vi "S4GUI.vi"() -> ()   [LabVIEW 2018] (continued)
        n3145 = call-dynamic "Read AcquisitionA.vi"("error in (no error)"=w7567, "S4ACS_GUI in"=w7556) -> ("error out"=w7581:errorcluster, "Acquisition.lvclass"=w7582:refnum<class "Acquisition.lvclass">)  [unwired: 7 in, 1 out]
        n3146 = call "Read AcquisitionB.vi"("error in (no error)"=w7567, "S4ACS_GUI in"=w7556) -> ("error out"=w7579:errorcluster, "Acquisition.lvclass"=w7580:refnum<class "Acquisition.lvclass">)  [unwired: 7 in, 1 out]
        n3147 = call-dynamic "Read AcquisitionD.vi"("error in (no error)"=w7567, "S4ACS_GUI in"=w7556) -> ("error out"=w7575:errorcluster, "Acquisition.lvclass"=w7576:refnum<class "Acquisition.lvclass">)  [unwired: 7 in, 1 out]
        n3148 = call "Read connection.vi"("error in (no error)"=w7578, "Server in"=w7577) -> ("error out"=w7584:errorcluster, "connection"=w7583:bool, "Server out"=w7585:refnum<class "Acquisition.lvclass">)  [unwired: 7 in]
        n3149 = call "Read connection.vi"("error in (no error)"=w7579, "Server in"=w7580) -> ("error out"=w7587:errorcluster, "connection"=w7586:bool, "Server out"=w7588:refnum<class "Acquisition.lvclass">)  [unwired: 7 in]
        n3150 = call "Read connection.vi"("error in (no error)"=w7575, "Server in"=w7576) -> ("error out"=w7564:errorcluster, "connection"=w7565:bool, "Server out"=w7566:refnum<class "Acquisition.lvclass">)  [unwired: 7 in]
        n3151 = call "Read connection.vi"("error in (no error)"=w7581, "Server in"=w7582) -> ("error out"=w7590:errorcluster, "connection"=w7589:bool, "Server out"=w7591:refnum<class "Acquisition.lvclass">)  [unwired: 7 in]
        n3152 = case shown="True" w7583 {
          tunnel: w7585 -> [w7758 w7763]
          tunnel: w7584 -> [w7757 w7762]
          tunnel: [w7758 w7761] -> w7570
          tunnel: [w7757 w7760] -> w7569
          tunnel: w7563 -> [_ w7759]
          frame False {
          }
          frame True {
            # "nome do arquivo .cfg"
            # "seção no arquivo .cfg"
            n3153 = call-dynamic "Read Channel.vi"("error in (no error)"=w7762, "Acquisition in"=w7763) -> ("error out"=w7767:errorcluster, "Channel.lvclass"=w7766:refnum<class "Channel.lvclass">, "Acquisition out"=w7765:refnum<class "Acquisition.lvclass">)  [unwired: 7 in]
            n3154 = call-dynamic "Read Interface.vi"("error in (no error)"=w7767, "Channel in"=w7766) -> ("error out"=w7774:errorcluster, "Interface.lvclass"=w7775:refnum<class "Interface.lvclass">, "Channel out"=w7764:refnum<class "Channel.lvclass">)  [unwired: 7 in]
            n3155 = call-dynamic "Get CCD_Config.vi"("error in (no error)"=w7774, "Interface in"=w7775) -> ("error out"=w7772:errorcluster, "output cluster"=w7771:T24, "Interface out"=w7776:refnum<class "Interface.lvclass">)  [unwired: 7 in]
            n3156 = Bundle By Name(cluster=w7771, "TRIGGER_MODE"=w7759) -> (w7773:T24)
            n3157 = call-dynamic "Set CCD_Config.vi"("error in (no error)"=w7772, "input cluster"=w7773, "Interface in"=w7776) -> ("error out"=w7770:errorcluster, "Interface out"=w7777:refnum<class "Interface.lvclass">)  [unwired: 7 in]
            n3158 = Flatten To String(anything=w7773, error in (no error)=w7770) -> (data string=w7768:string, error out=w7769:errorcluster)  [unwired: 2 in, 1 out]
            n3159 = call "Write flatted cluster.vi"("error in (no error)"=w7769, "flatted cluster"=w7768, "Interface in"=w7777) -> ("error out"=w7779:errorcluster, "Interface out"=w7778:refnum<class "Interface.lvclass">)  [unwired: 7 in]
            n3160 = call-dynamic "Write Interface.vi"("error in (no error)"=w7779, "Interface.lvclass"=w7778, "Channel in"=w7764) -> ("error out"=w7785:errorcluster, "Channel out"=w7786:refnum<class "Channel.lvclass">)  [unwired: 7 in]
            n3161 = call "Write section_name.vi"("error in (no error)"=w7785, "section_name"="CCD_ACS3", "Channel in"=w7786) -> ("error out"=w7783:errorcluster, "Channel out"=w7789:refnum<class "Channel.lvclass">)  [unwired: 7 in]
            n3162 = call-dynamic "save config.vi"("error in (no error)"=w7783, "file config"="lastsaved.cfg", "Channel in"=w7789) -> ("error out"=w7784:errorcluster, "Channel out"=w7790:refnum<class "Channel.lvclass">)  [unwired: 7 in]
            n3163 = call-dynamic "Read State Machine.vi"("error in (no error)"=w7784, "Device in"=w7790) -> ("error out"=w7780:errorcluster, "State Machine.lvclass"=w7792:refnum<class "State Machine.lvclass">, "Device out"=w7791:refnum<class "Channel.lvclass">)  [unwired: 7 in]
            n3164 = call-dynamic "Write State.vi"("error in (no error)"=w7780, "State"=60, "State Machine in"=w7792) -> ("error out"=w7781:errorcluster, "State Machine out"=w7793:refnum<class "State Machine.lvclass">)  [unwired: 7 in]
            n3165 = call-dynamic "Write State Machine.vi"("error in (no error)"=w7781, "State Machine.lvclass"=w7793, "Device in"=w7791) -> ("error out"=w7795:errorcluster, "Device out"=w7794:refnum<class "Channel.lvclass">)  [unwired: 7 in]
            n3166 = call-dynamic "Write Channel.vi"("error in (no error)"=w7795, "Channel.lvclass"=w7794, "Acquisition in"=w7765) -> ("error out"=w7760:errorcluster, "Acquisition out"=w7761:refnum<class "Acquisition.lvclass">)  [unwired: 7 in]
          }
        }
        n3167 = case shown="True" w7565 {
          tunnel: w7566 -> [w7719 w7724]
          tunnel: w7564 -> [w7718 w7723]
          tunnel: w7563 -> [_ w7722]
          tunnel: [w7719 w7721] -> w7562
          tunnel: [w7718 w7720] -> w7561
          frame False {
          }
          frame True {
            # "nome do arquivo .cfg"
            # "seção no arquivo .cfg"
            n3168 = call-dynamic "Read Channel.vi"("error in (no error)"=w7723, "Acquisition in"=w7724) -> ("error out"=w7753:errorcluster, "Channel.lvclass"=w7754:refnum<class "Channel.lvclass">, "Acquisition out"=w7755:refnum<class "Acquisition.lvclass">)  [unwired: 7 in]
            n3169 = call-dynamic "Read Interface.vi"("error in (no error)"=w7753, "Channel in"=w7754) -> ("error out"=w7746:errorcluster, "Interface.lvclass"=w7745:refnum<class "Interface.lvclass">, "Channel out"=w7756:refnum<class "Channel.lvclass">)  [unwired: 7 in]
            n3170 = call-dynamic "Get CCD_Config.vi"("error in (no error)"=w7746, "Interface in"=w7745) -> ("error out"=w7748:errorcluster, "output cluster"=w7749:T24, "Interface out"=w7744:refnum<class "Interface.lvclass">)  [unwired: 7 in]
            n3171 = Bundle By Name(cluster=w7749, "TRIGGER_MODE"=w7722) -> (w7747:T24)
            n3172 = call-dynamic "Set CCD_Config.vi"("error in (no error)"=w7748, "input cluster"=w7747, "Interface in"=w7744) -> ("error out"=w7750:errorcluster, "Interface out"=w7743:refnum<class "Interface.lvclass">)  [unwired: 7 in]
            n3173 = Flatten To String(anything=w7747, error in (no error)=w7750) -> (data string=w7752:string, error out=w7751:errorcluster)  [unwired: 2 in, 1 out]
            n3174 = call "Write flatted cluster.vi"("error in (no error)"=w7751, "flatted cluster"=w7752, "Interface in"=w7743) -> ("error out"=w7741:errorcluster, "Interface out"=w7742:refnum<class "Interface.lvclass">)  [unwired: 7 in]
            n3175 = call-dynamic "Write Interface.vi"("error in (no error)"=w7741, "Interface.lvclass"=w7742, "Channel in"=w7756) -> ("error out"=w7735:errorcluster, "Channel out"=w7734:refnum<class "Channel.lvclass">)  [unwired: 7 in]
            n3176 = call "Write section_name.vi"("error in (no error)"=w7735, "section_name"="CCD_ACS4", "Channel in"=w7734) -> ("error out"=w7737:errorcluster, "Channel out"=w7731:refnum<class "Channel.lvclass">)  [unwired: 7 in]
            n3177 = call-dynamic "save config.vi"("error in (no error)"=w7737, "file config"="lastsaved.cfg", "Channel in"=w7731) -> ("error out"=w7736:errorcluster, "Channel out"=w7730:refnum<class "Channel.lvclass">)  [unwired: 7 in]
            n3178 = call-dynamic "Read State Machine.vi"("error in (no error)"=w7736, "Device in"=w7730) -> ("error out"=w7740:errorcluster, "State Machine.lvclass"=w7728:refnum<class "State Machine.lvclass">, "Device out"=w7729:refnum<class "Channel.lvclass">)  [unwired: 7 in]
            n3179 = call-dynamic "Write State.vi"("error in (no error)"=w7740, "State"=60, "State Machine in"=w7728) -> ("error out"=w7739:errorcluster, "State Machine out"=w7727:refnum<class "State Machine.lvclass">)  [unwired: 7 in]
            n3180 = call-dynamic "Write State Machine.vi"("error in (no error)"=w7739, "State Machine.lvclass"=w7727, "Device in"=w7729) -> ("error out"=w7725:errorcluster, "Device out"=w7726:refnum<class "Channel.lvclass">)  [unwired: 7 in]
            n3181 = call-dynamic "Write Channel.vi"("error in (no error)"=w7725, "Channel.lvclass"=w7726, "Acquisition in"=w7755) -> ("error out"=w7720:errorcluster, "Acquisition out"=w7721:refnum<class "Acquisition.lvclass">)  [unwired: 7 in]
          }
        }
        n3182 = case shown="True" w7586 {
          tunnel: w7588 -> [w7797 w7802]
          tunnel: w7587 -> [w7796 w7801]
          tunnel: [w7797 w7800] -> w7572
          tunnel: [w7796 w7799] -> w7571
          tunnel: w7563 -> [_ w7798]
          frame False {
          }
          frame True {
            # "nome do arquivo .cfg"
            # "seção no arquivo .cfg"
            n3183 = call-dynamic "Read Channel.vi"("error in (no error)"=w7801, "Acquisition in"=w7802) -> ("error out"=w7806:errorcluster, "Channel.lvclass"=w7805:refnum<class "Channel.lvclass">, "Acquisition out"=w7804:refnum<class "Acquisition.lvclass">)  [unwired: 7 in]
            n3184 = call-dynamic "Read Interface.vi"("error in (no error)"=w7806, "Channel in"=w7805) -> ("error out"=w7813:errorcluster, "Interface.lvclass"=w7814:refnum<class "Interface.lvclass">, "Channel out"=w7803:refnum<class "Channel.lvclass">)  [unwired: 7 in]
            n3185 = call-dynamic "Get CCD_Config.vi"("error in (no error)"=w7813, "Interface in"=w7814) -> ("error out"=w7811:errorcluster, "output cluster"=w7810:T24, "Interface out"=w7815:refnum<class "Interface.lvclass">)  [unwired: 7 in]
            n3186 = Bundle By Name(cluster=w7810, "TRIGGER_MODE"=w7798) -> (w7812:T24)
            n3187 = call-dynamic "Set CCD_Config.vi"("error in (no error)"=w7811, "input cluster"=w7812, "Interface in"=w7815) -> ("error out"=w7809:errorcluster, "Interface out"=w7816:refnum<class "Interface.lvclass">)  [unwired: 7 in]
            n3188 = Flatten To String(anything=w7812, error in (no error)=w7809) -> (data string=w7807:string, error out=w7808:errorcluster)  [unwired: 2 in, 1 out]
            n3189 = call "Write flatted cluster.vi"("error in (no error)"=w7808, "flatted cluster"=w7807, "Interface in"=w7816) -> ("error out"=w7818:errorcluster, "Interface out"=w7817:refnum<class "Interface.lvclass">)  [unwired: 7 in]
            n3190 = call-dynamic "Write Interface.vi"("error in (no error)"=w7818, "Interface.lvclass"=w7817, "Channel in"=w7803) -> ("error out"=w7824:errorcluster, "Channel out"=w7825:refnum<class "Channel.lvclass">)  [unwired: 7 in]
            n3191 = call "Write section_name.vi"("error in (no error)"=w7824, "section_name"="CCD_ACS2", "Channel in"=w7825) -> ("error out"=w7822:errorcluster, "Channel out"=w7828:refnum<class "Channel.lvclass">)  [unwired: 7 in]
            n3192 = call-dynamic "save config.vi"("error in (no error)"=w7822, "file config"="lastsaved.cfg", "Channel in"=w7828) -> ("error out"=w7823:errorcluster, "Channel out"=w7829:refnum<class "Channel.lvclass">)  [unwired: 7 in]
            n3193 = call-dynamic "Read State Machine.vi"("error in (no error)"=w7823, "Device in"=w7829) -> ("error out"=w7819:errorcluster, "State Machine.lvclass"=w7831:refnum<class "State Machine.lvclass">, "Device out"=w7830:refnum<class "Channel.lvclass">)  [unwired: 7 in]
            n3194 = call-dynamic "Write State.vi"("error in (no error)"=w7819, "State"=60, "State Machine in"=w7831) -> ("error out"=w7820:errorcluster, "State Machine out"=w7832:refnum<class "State Machine.lvclass">)  [unwired: 7 in]
            n3195 = call-dynamic "Write State Machine.vi"("error in (no error)"=w7820, "State Machine.lvclass"=w7832, "Device in"=w7830) -> ("error out"=w7834:errorcluster, "Device out"=w7833:refnum<class "Channel.lvclass">)  [unwired: 7 in]
            n3196 = call-dynamic "Write Channel.vi"("error in (no error)"=w7834, "Channel.lvclass"=w7833, "Acquisition in"=w7804) -> ("error out"=w7799:errorcluster, "Acquisition out"=w7800:refnum<class "Acquisition.lvclass">)  [unwired: 7 in]
          }
        }
        n3197 = case shown="True" w7589 {
          tunnel: [w7835 w7869] -> w7573
          tunnel: [w7836 w7868] -> w7574
          tunnel: w7591 -> [w7836 w7839]
          tunnel: w7590 -> [w7835 w7838]
          tunnel: w7563 -> [_ w7837]
          frame False {
          }
          frame True {
            # "nome do arquivo .cfg"
            # "seção no arquivo .cfg"
            n3198 = call-dynamic "Read Channel.vi"("error in (no error)"=w7838, "Acquisition in"=w7839) -> ("error out"=w7870:errorcluster, "Channel.lvclass"=w7871:refnum<class "Channel.lvclass">, "Acquisition out"=w7872:refnum<class "Acquisition.lvclass">)  [unwired: 7 in]
            n3199 = call-dynamic "Read Interface.vi"("error in (no error)"=w7870, "Channel in"=w7871) -> ("error out"=w7861:errorcluster, "Interface.lvclass"=w7860:refnum<class "Interface.lvclass">, "Channel out"=w7873:refnum<class "Channel.lvclass">)  [unwired: 7 in]
            n3200 = call-dynamic "Get CCD_Config.vi"("error in (no error)"=w7861, "Interface in"=w7860) -> ("error out"=w7863:errorcluster, "output cluster"=w7864:T24, "Interface out"=w7859:refnum<class "Interface.lvclass">)  [unwired: 7 in]
            n3201 = Bundle By Name(cluster=w7864, "TRIGGER_MODE"=w7837) -> (w7862:T24)
            n3202 = call-dynamic "Set CCD_Config.vi"("error in (no error)"=w7863, "input cluster"=w7862, "Interface in"=w7859) -> ("error out"=w7865:errorcluster, "Interface out"=w7858:refnum<class "Interface.lvclass">)  [unwired: 7 in]
            n3203 = Flatten To String(anything=w7862, error in (no error)=w7865) -> (data string=w7867:string, error out=w7866:errorcluster)  [unwired: 2 in, 1 out]
            n3204 = call "Write flatted cluster.vi"("error in (no error)"=w7866, "flatted cluster"=w7867, "Interface in"=w7858) -> ("error out"=w7856:errorcluster, "Interface out"=w7857:refnum<class "Interface.lvclass">)  [unwired: 7 in]
            n3205 = call-dynamic "Write Interface.vi"("error in (no error)"=w7856, "Interface.lvclass"=w7857, "Channel in"=w7873) -> ("error out"=w7851:errorcluster, "Channel out"=w7850:refnum<class "Channel.lvclass">)  [unwired: 7 in]
            n3206 = call "Write section_name.vi"("error in (no error)"=w7851, "section_name"="CCD_ACS1", "Channel in"=w7850) -> ("error out"=w7852:errorcluster, "Channel out"=w7847:refnum<class "Channel.lvclass">)  [unwired: 7 in]
            n3207 = call-dynamic "save config.vi"("error in (no error)"=w7852, "file config"="lastsaved.cfg", "Channel in"=w7847) -> ("error out"=w7840:errorcluster, "Channel out"=w7841:refnum<class "Channel.lvclass">)  [unwired: 7 in]
            n3208 = call-dynamic "Read State Machine.vi"("error in (no error)"=w7840, "Device in"=w7841) -> ("error out"=w7855:errorcluster, "State Machine.lvclass"=w7845:refnum<class "State Machine.lvclass">, "Device out"=w7846:refnum<class "Channel.lvclass">)  [unwired: 7 in]
            n3209 = call-dynamic "Write State.vi"("error in (no error)"=w7855, "State"=60, "State Machine in"=w7845) -> ("error out"=w7854:errorcluster, "State Machine out"=w7844:refnum<class "State Machine.lvclass">)  [unwired: 7 in]
            n3210 = call-dynamic "Write State Machine.vi"("error in (no error)"=w7854, "State Machine.lvclass"=w7844, "Device in"=w7846) -> ("error out"=w7842:errorcluster, "Device out"=w7843:refnum<class "Channel.lvclass">)  [unwired: 7 in]
            n3211 = call-dynamic "Write Channel.vi"("error in (no error)"=w7842, "Channel.lvclass"=w7843, "Acquisition in"=w7872) -> ("error out"=w7869:errorcluster, "Acquisition out"=w7868:refnum<class "Acquisition.lvclass">)  [unwired: 7 in]
          }
        }
        n3212 = call-dynamic "Write AcquisitionA.vi"("error in (no error)"=w7573, "Acquisition.lvclass"=w7574, "S4ACS_GUI in"=w7556) -> ("error out"=w7560:errorcluster, "S4ACS_GUI out"=w7555:refnum<class "S4GUI.lvclass">)  [unwired: 7 in]
        n3213 = call "Write AcquisitionB.vi"("error in (no error)"=w7571, "Acquisition.lvclass"=w7572, "S4ACS_GUI in"=w7555) -> ("error out"=w7559:errorcluster, "S4ACS_GUI out"=w7554:refnum<class "S4GUI.lvclass">)  [unwired: 7 in]
        n3214 = call-dynamic "Write AcquisitionC.vi"("error in (no error)"=w7569, "Acquisition.lvclass"=w7570, "S4ACS_GUI in"=w7554) -> ("error out"=w7558:errorcluster, "S4ACS_GUI out"=w7553:refnum<class "S4GUI.lvclass">)  [unwired: 7 in]
        n3215 = call-dynamic "Write AcquisitionD.vi"("error in (no error)"=w7561, "Acquisition.lvclass"=w7562, "S4ACS_GUI in"=w7553) -> ("error out"=w7557:errorcluster, "S4ACS_GUI out"=w7536:refnum<class "S4GUI.lvclass">)  [unwired: 7 in]
        n3216 = Merge Errors(w7560, w7559, w7558, w7557) -> (w7533:errorcluster)
        n3217 = call "Read Instrument.lvclass.vi"("error in (no error)"=w7533, "S4ACS_GUI in"=w7536) -> ("error out"=w7541:errorcluster, "Instrument.lvclass"=w7540:refnum<class "Instrument.lvclass">, "S4ACS_GUI out"=w7537:refnum<class "S4GUI.lvclass">)  [unwired: 7 in]
        n3218 = call "Read ASEL.vi"("error in (no error)"=w7541, "Instrument in"=w7540) -> ("error out"=w7549:errorcluster, "Opt_Selector.lvclass"=w7548:refnum<class "Opt_Selector.lvclass">, "Instrument out"=w7547:refnum<class "Instrument.lvclass">)  [unwired: 7 in]
        n3219 = call "Read target name.vi"("error in (no error)"=w7549, "Optics in"=w7548) -> ("error out"=w7545:errorcluster, "target name"=w7544:string, "Optics out"=w7546:refnum<class "Opt_Selector.lvclass">)  [unwired: 7 in]
        n3220 = call "Write ASEL.vi"("error in (no error)"=w7545, "Opt_Selector.lvclass"=w7546, "Instrument in"=w7547) -> ("error out"=w7543:errorcluster, "Instrument out"=w7539:refnum<class "Instrument.lvclass">)  [unwired: 7 in]
        n3221 = case shown="\"ON\"" w7544 {
          tunnel: w7543 -> [w7694 w7705]
          tunnel: [w7694 w7701] -> w7542
          tunnel: w7539 -> [w7693 w7706]
          tunnel: [w7693 w7702] -> w7538
          frame Default {
          }
          frame "ON" {
            n3222 = call "Read WPROT.vi"("error in (no error)"=w7705, "Instrument in"=w7706) -> ("error out"=w7697:errorcluster, "Opt_Selector.lvclass"=w7704:refnum<class "Opt_Selector.lvclass">, "Instrument out"=w7703:refnum<class "Instrument.lvclass">)  [unwired: 7 in]
            n3223 = call-dynamic "Read sequencia.vi"("error in (no error)"=w7697, "Opt_Selector in"=w7704) -> ("error out"=w7696:errorcluster, "sequencia"=w7700:u16, "Opt_Selector out"=w7699:refnum<class "Opt_Selector.lvclass">)  [unwired: 7 in]
            n3224 = case shown="0" w7700 {
              tunnel: w7699 -> [w7708 w7717]
              tunnel: [w7708 w7713] -> w7698
              tunnel: w7696 -> [w7707 w7716]
              tunnel: [w7707 w7711] -> w7695
              frame Default {
              }
              frame 0 {
                n3225 = call-dynamic "Write sequencia.vi"("error in (no error)"=w7716, "sequencia"=u16 1, "Opt_Selector in"=w7717) -> ("error out"=w7712:errorcluster, "Opt_Selector out"=w7714:refnum<class "Opt_Selector.lvclass">)  [unwired: 7 in]
                n3226 = local write "P0"(TRUE ("P0")) -> ()
                n3227 = call-dynamic "Write sequencia_ant.vi"("error in (no error)"=w7712, "sequencia_ant"=u16 1, "Opt_Selector in"=w7714) -> ("error out"=w7711:errorcluster, "Opt_Selector out"=w7713:refnum<class "Opt_Selector.lvclass">)  [unwired: 7 in]
              }
            }
            n3228 = call "Write WPROT.vi"("error in (no error)"=w7695, "Opt_Selector.lvclass"=w7698, "Instrument in"=w7703) -> ("error out"=w7701:errorcluster, "Instrument out"=w7702:refnum<class "Instrument.lvclass">)  [unwired: 7 in]
          }
        }
        n3229 = call "Write Instrument.lvclass.vi"("error in (no error)"=w7542, "Instrument.lvclass"=w7538, "S4ACS_GUI in"=w7537) -> ("error out"=w7534:errorcluster, "S4ACS_GUI out"=w7535:refnum<class "S4GUI.lvclass">)  [unwired: 7 in]
      }
      event "Init mode": Value Change {
        n3230 = event-data() -> ()  [unwired: 1 in, 4 out]
        n3231 = call-dynamic "Read Obs_state.vi"("error in (no error)"=w7929, "S4ACS_GUI in"=w7930) -> ("error out"=w7923:errorcluster, "Obs_state"=w7925:u32, "S4ACS_GUI out"=w7926:refnum<class "S4GUI.lvclass">)  [unwired: 7 in]
        n3232 = In Range and Coerce(upper limit=u32 226, x=w7925, lower limit=u32 220 ("upper limit")) -> (In Range?=w7924:bool)  [unwired: 1 out]
        n3233 = case shown="False" w7924 {
          tunnel: [w7936 w7944] -> w7932
          tunnel: [w7935 w7942] -> w7931
          tunnel: w7923 -> [w7934 w7943]
          tunnel: w7926 -> [w7933 w7945]
          frame False {
            n3234 = call-dynamic "Write sync.vi"("error in (no error)"=w7934, "sync"=TRUE, "S4ACS_GUI in"=w7933) -> ("error out"=w7938:errorcluster, "S4ACS_GUI out"=w7937:refnum<class "S4GUI.lvclass">)  [unwired: 7 in]
            n3235 = call-dynamic "Write Obs_state.vi"("error in (no error)"=w7938, "Obs_state"=u32 220, "S4ACS_GUI in"=w7937) -> ("error out"=w7935:errorcluster, "S4ACS_GUI out"=w7936:refnum<class "S4GUI.lvclass">)  [unwired: 7 in]
          }
          frame True {
            n3236 = call-dynamic "Write Obs_state.vi"("error in (no error)"=w7943, "Obs_state"=u32 0, "S4ACS_GUI in"=w7945) -> ("error out"=w7942:errorcluster, "S4ACS_GUI out"=w7944:refnum<class "S4GUI.lvclass">)  [unwired: 7 in]
          }
        }
      }
      event "Set PCS": Value Change {
        n3237 = event-data() -> ()  [unwired: 1 in, 4 out]
        n3238 = call "Read Instrument.lvclass.vi"("error in (no error)"=w7964, "S4ACS_GUI in"=w7965) -> ("error out"=w7962:errorcluster, "Instrument.lvclass"=w7963:refnum<class "Instrument.lvclass">, "S4ACS_GUI out"=w7951:refnum<class "S4GUI.lvclass">)  [unwired: 7 in]
        n3239 = call "Read CALW.vi"("error in (no error)"=w7962, "Instrument in"=w7963) -> ("error out"=w7959:errorcluster, "Opt_Selector.lvclass"=w7961:refnum<class "Opt_Selector.lvclass">, "Instrument out"=w7953:refnum<class "Instrument.lvclass">)  [unwired: 7 in]
        n3240 = call-dynamic "Read State Machine.vi"("error in (no error)"=w7959, "Device in"=w7961) -> ("error out"=w7958:errorcluster, "State Machine.lvclass"=w7949:refnum<class "State Machine.lvclass">, "Device out"=w7955:refnum<class "Opt_Selector.lvclass">)  [unwired: 7 in]
        n3241 = call "Next State.vi"("error in (no error)"=w7958, "New_State"=1, "State Machine in"=w7949) -> ("error out"=w7957:errorcluster, "State Machine out"=w7956:refnum<class "State Machine.lvclass">)  [unwired: 7 in]
        n3242 = call-dynamic "Write State Machine.vi"("error in (no error)"=w7957, "State Machine.lvclass"=w7956, "Device in"=w7955) -> ("error out"=w7952:errorcluster, "Device out"=w7954:refnum<class "Opt_Selector.lvclass">)  [unwired: 7 in]
        n3243 = call "Write CALW.vi"("error in (no error)"=w7952, "Opt_Selector.lvclass"=w7954, "Instrument in"=w7953) -> ("error out"=w7947:errorcluster, "Instrument out"=w7948:refnum<class "Instrument.lvclass">)  [unwired: 7 in]
        n3244 = call "Write Instrument.lvclass.vi"("error in (no error)"=w7947, "Instrument.lvclass"=w7948, "S4ACS_GUI in"=w7951) -> ("error out"=w7950:errorcluster, "S4ACS_GUI out"=w7946:refnum<class "S4GUI.lvclass">)  [unwired: 7 in]
      }
      event "WPSEL_stop": Value Change {
        n3245 = event-data() -> ()  [unwired: 1 in, 4 out]
        n3246 = call "Read Instrument.lvclass.vi"("error in (no error)"=w7984, "S4ACS_GUI in"=w7985) -> ("error out"=w7982:errorcluster, "Instrument.lvclass"=w7983:refnum<class "Instrument.lvclass">, "S4ACS_GUI out"=w7969:refnum<class "S4GUI.lvclass">)  [unwired: 7 in]
        n3247 = call "Read WPSEL.vi"("error in (no error)"=w7982, "Instrument in"=w7983) -> ("error out"=w7978:errorcluster, "Opt_Selector.lvclass"=w7981:refnum<class "Opt_Selector.lvclass">, "Instrument out"=w7972:refnum<class "Instrument.lvclass">)  [unwired: 7 in]
        n3248 = call-dynamic "Read State Machine.vi"("error in (no error)"=w7978, "Device in"=w7981) -> ("error out"=w7977:errorcluster, "State Machine.lvclass"=w7980:refnum<class "State Machine.lvclass">, "Device out"=w7974:refnum<class "Opt_Selector.lvclass">)  [unwired: 7 in]
        n3249 = call "Next State.vi"("error in (no error)"=w7977, "New_State"=10, "State Machine in"=w7980) -> ("error out"=w7976:errorcluster, "State Machine out"=w7975:refnum<class "State Machine.lvclass">)  [unwired: 7 in]
        n3250 = call-dynamic "Write State Machine.vi"("error in (no error)"=w7976, "State Machine.lvclass"=w7975, "Device in"=w7974) -> ("error out"=w7971:errorcluster, "Device out"=w7973:refnum<class "Opt_Selector.lvclass">)  [unwired: 7 in]
        n3251 = call "Write WPSEL.vi"("error in (no error)"=w7971, "Opt_Selector.lvclass"=w7973, "Instrument in"=w7972) -> ("error out"=w7968:errorcluster, "Instrument out"=w7970:refnum<class "Instrument.lvclass">)  [unwired: 7 in]
        n3252 = call "Write Instrument.lvclass.vi"("error in (no error)"=w7968, "Instrument.lvclass"=w7970, "S4ACS_GUI in"=w7969) -> ("error out"=w7967:errorcluster, "S4ACS_GUI out"=w7966:refnum<class "S4GUI.lvclass">)  [unwired: 7 in]
      }
      event "WPSEL_init": Value Change {
        n3253 = event-data() -> ()  [unwired: 1 in, 4 out]
        n3254 = call "Read Instrument.lvclass.vi"("error in (no error)"=w8004, "S4ACS_GUI in"=w8005) -> ("error out"=w8002:errorcluster, "Instrument.lvclass"=w8003:refnum<class "Instrument.lvclass">, "S4ACS_GUI out"=w7989:refnum<class "S4GUI.lvclass">)  [unwired: 7 in]
        n3255 = call "Read WPSEL.vi"("error in (no error)"=w8002, "Instrument in"=w8003) -> ("error out"=w7998:errorcluster, "Opt_Selector.lvclass"=w8001:refnum<class "Opt_Selector.lvclass">, "Instrument out"=w7992:refnum<class "Instrument.lvclass">)  [unwired: 7 in]
        n3256 = call-dynamic "Read State Machine.vi"("error in (no error)"=w7998, "Device in"=w8001) -> ("error out"=w7997:errorcluster, "State Machine.lvclass"=w8000:refnum<class "State Machine.lvclass">, "Device out"=w7994:refnum<class "Opt_Selector.lvclass">)  [unwired: 7 in]
        n3257 = call "Next State.vi"("error in (no error)"=w7997, "New_State"=30, "State Machine in"=w8000) -> ("error out"=w7996:errorcluster, "State Machine out"=w7995:refnum<class "State Machine.lvclass">)  [unwired: 7 in]
        n3258 = call-dynamic "Write State Machine.vi"("error in (no error)"=w7996, "State Machine.lvclass"=w7995, "Device in"=w7994) -> ("error out"=w7991:errorcluster, "Device out"=w7993:refnum<class "Opt_Selector.lvclass">)  [unwired: 7 in]
        n3259 = call "Write WPSEL.vi"("error in (no error)"=w7991, "Opt_Selector.lvclass"=w7993, "Instrument in"=w7992) -> ("error out"=w7988:errorcluster, "Instrument out"=w7990:refnum<class "Instrument.lvclass">)  [unwired: 7 in]
        n3260 = call "Write Instrument.lvclass.vi"("error in (no error)"=w7988, "Instrument.lvclass"=w7990, "S4ACS_GUI in"=w7989) -> ("error out"=w7987:errorcluster, "S4ACS_GUI out"=w7986:refnum<class "S4GUI.lvclass">)  [unwired: 7 in]
      }
      event "GMIR_target": Value Change {
        n3261 = event-data() -> ("NewVal"=w8015:dbl)  [unwired: 1 in, 3 out]
        n3262 = call "Read Instrument.lvclass.vi"("error in (no error)"=w8019, "S4ACS_GUI in"=w8020) -> ("error out"=w8017:errorcluster, "Instrument.lvclass"=w8018:refnum<class "Instrument.lvclass">, "S4ACS_GUI out"=w8009:refnum<class "S4GUI.lvclass">)  [unwired: 7 in]
        n3263 = call "Read GMIR.vi"("error in (no error)"=w8017, "Instrument in"=w8018) -> ("error out"=w8014:errorcluster, "Opt_Continuous.lvclass"=w8016:refnum<class "Opt_Continuous.lvclass">, "Instrument out"=w8012:refnum<class "Instrument.lvclass">)  [unwired: 7 in]
        n3264 = call "Write target.vi"("error in (no error)"=w8014, "target"=w8015, "Optics in"=w8016) -> ("error out"=w8011:errorcluster, "Optics out"=w8013:refnum<class "Opt_Continuous.lvclass">)  [unwired: 7 in]
        n3265 = call "Write GMIR.vi"("error in (no error)"=w8011, "Opt_Continuous.lvclass"=w8013, "Instrument in"=w8012) -> ("error out"=w8008:errorcluster, "Instrument out"=w8010:refnum<class "Instrument.lvclass">)  [unwired: 7 in]
        n3266 = call "Write Instrument.lvclass.vi"("error in (no error)"=w8008, "Instrument.lvclass"=w8010, "S4ACS_GUI in"=w8009) -> ("error out"=w8007:errorcluster, "S4ACS_GUI out"=w8006:refnum<class "S4GUI.lvclass">)  [unwired: 7 in]
      }
      event "GMIR_set": Value Change {
        n3267 = event-data() -> ()  [unwired: 1 in, 4 out]
        n3268 = call "Read Instrument.lvclass.vi"("error in (no error)"=w8039, "S4ACS_GUI in"=w8040) -> ("error out"=w8037:errorcluster, "Instrument.lvclass"=w8038:refnum<class "Instrument.lvclass">, "S4ACS_GUI out"=w8026:refnum<class "S4GUI.lvclass">)  [unwired: 7 in]
        n3269 = call "Read GMIR.vi"("error in (no error)"=w8037, "Instrument in"=w8038) -> ("error out"=w8034:errorcluster, "Opt_Continuous.lvclass"=w8036:refnum<class "Opt_Continuous.lvclass">, "Instrument out"=w8028:refnum<class "Instrument.lvclass">)  [unwired: 7 in]
        n3270 = call-dynamic "Read State Machine.vi"("error in (no error)"=w8034, "Device in"=w8036) -> ("error out"=w8033:errorcluster, "State Machine.lvclass"=w8024:refnum<class "State Machine.lvclass">, "Device out"=w8030:refnum<class "Opt_Continuous.lvclass">)  [unwired: 7 in]
        n3271 = call "Next State.vi"("error in (no error)"=w8033, "New_State"=1, "State Machine in"=w8024) -> ("error out"=w8032:errorcluster, "State Machine out"=w8031:refnum<class "State Machine.lvclass">)  [unwired: 7 in]
        n3272 = call-dynamic "Write State Machine.vi"("error in (no error)"=w8032, "State Machine.lvclass"=w8031, "Device in"=w8030) -> ("error out"=w8027:errorcluster, "Device out"=w8029:refnum<class "Opt_Continuous.lvclass">)  [unwired: 7 in]
        n3273 = call "Write GMIR.vi"("error in (no error)"=w8027, "Opt_Continuous.lvclass"=w8029, "Instrument in"=w8028) -> ("error out"=w8021:errorcluster, "Instrument out"=w8022:refnum<class "Instrument.lvclass">)  [unwired: 7 in]
        n3274 = call "Write Instrument.lvclass.vi"("error in (no error)"=w8021, "Instrument.lvclass"=w8022, "S4ACS_GUI in"=w8026) -> ("error out"=w8025:errorcluster, "S4ACS_GUI out"=w8023:refnum<class "S4GUI.lvclass">)  [unwired: 7 in]
      }
      event "GMIR_stop": Value Change {
        n3275 = event-data() -> ()  [unwired: 1 in, 4 out]
        n3276 = call "Read Instrument.lvclass.vi"("error in (no error)"=w8059, "S4ACS_GUI in"=w8060) -> ("error out"=w8057:errorcluster, "Instrument.lvclass"=w8058:refnum<class "Instrument.lvclass">, "S4ACS_GUI out"=w8044:refnum<class "S4GUI.lvclass">)  [unwired: 7 in]
        n3277 = call "Read GMIR.vi"("error in (no error)"=w8057, "Instrument in"=w8058) -> ("error out"=w8053:errorcluster, "Opt_Continuous.lvclass"=w8056:refnum<class "Opt_Continuous.lvclass">, "Instrument out"=w8047:refnum<class "Instrument.lvclass">)  [unwired: 7 in]
        n3278 = call-dynamic "Read State Machine.vi"("error in (no error)"=w8053, "Device in"=w8056) -> ("error out"=w8052:errorcluster, "State Machine.lvclass"=w8055:refnum<class "State Machine.lvclass">, "Device out"=w8049:refnum<class "Opt_Continuous.lvclass">)  [unwired: 7 in]
        n3279 = call "Next State.vi"("error in (no error)"=w8052, "New_State"=10, "State Machine in"=w8055) -> ("error out"=w8051:errorcluster, "State Machine out"=w8050:refnum<class "State Machine.lvclass">)  [unwired: 7 in]
        n3280 = call-dynamic "Write State Machine.vi"("error in (no error)"=w8051, "State Machine.lvclass"=w8050, "Device in"=w8049) -> ("error out"=w8046:errorcluster, "Device out"=w8048:refnum<class "Opt_Continuous.lvclass">)  [unwired: 7 in]
        n3281 = call "Write GMIR.vi"("error in (no error)"=w8046, "Opt_Continuous.lvclass"=w8048, "Instrument in"=w8047) -> ("error out"=w8043:errorcluster, "Instrument out"=w8045:refnum<class "Instrument.lvclass">)  [unwired: 7 in]
        n3282 = call "Write Instrument.lvclass.vi"("error in (no error)"=w8043, "Instrument.lvclass"=w8045, "S4ACS_GUI in"=w8044) -> ("error out"=w8042:errorcluster, "S4ACS_GUI out"=w8041:refnum<class "S4GUI.lvclass">)  [unwired: 7 in]
      }
      event "GMIR_init": Value Change {
        n3283 = event-data() -> ()  [unwired: 1 in, 4 out]
        n3284 = call "Read Instrument.lvclass.vi"("error in (no error)"=w8079, "S4ACS_GUI in"=w8080) -> ("error out"=w8077:errorcluster, "Instrument.lvclass"=w8078:refnum<class "Instrument.lvclass">, "S4ACS_GUI out"=w8064:refnum<class "S4GUI.lvclass">)  [unwired: 7 in]
        n3285 = call "Read GMIR.vi"("error in (no error)"=w8077, "Instrument in"=w8078) -> ("error out"=w8073:errorcluster, "Opt_Continuous.lvclass"=w8076:refnum<class "Opt_Continuous.lvclass">, "Instrument out"=w8067:refnum<class "Instrument.lvclass">)  [unwired: 7 in]
        n3286 = call-dynamic "Read State Machine.vi"("error in (no error)"=w8073, "Device in"=w8076) -> ("error out"=w8072:errorcluster, "State Machine.lvclass"=w8075:refnum<class "State Machine.lvclass">, "Device out"=w8069:refnum<class "Opt_Continuous.lvclass">)  [unwired: 7 in]
        n3287 = call "Next State.vi"("error in (no error)"=w8072, "New_State"=30, "State Machine in"=w8075) -> ("error out"=w8071:errorcluster, "State Machine out"=w8070:refnum<class "State Machine.lvclass">)  [unwired: 7 in]
        n3288 = call-dynamic "Write State Machine.vi"("error in (no error)"=w8071, "State Machine.lvclass"=w8070, "Device in"=w8069) -> ("error out"=w8066:errorcluster, "Device out"=w8068:refnum<class "Opt_Continuous.lvclass">)  [unwired: 7 in]
        n3289 = call "Write GMIR.vi"("error in (no error)"=w8066, "Opt_Continuous.lvclass"=w8068, "Instrument in"=w8067) -> ("error out"=w8063:errorcluster, "Instrument out"=w8065:refnum<class "Instrument.lvclass">)  [unwired: 7 in]
        n3290 = call "Write Instrument.lvclass.vi"("error in (no error)"=w8063, "Instrument.lvclass"=w8065, "S4ACS_GUI in"=w8064) -> ("error out"=w8062:errorcluster, "S4ACS_GUI out"=w8061:refnum<class "S4GUI.lvclass">)  [unwired: 7 in]
      }
      event "GFOC_target": Value Change {
        n3291 = event-data() -> ("NewVal"=w8090:dbl)  [unwired: 1 in, 3 out]
        n3292 = call "Read Instrument.lvclass.vi"("error in (no error)"=w8094, "S4ACS_GUI in"=w8095) -> ("error out"=w8092:errorcluster, "Instrument.lvclass"=w8093:refnum<class "Instrument.lvclass">, "S4ACS_GUI out"=w8084:refnum<class "S4GUI.lvclass">)  [unwired: 7 in]
        n3293 = call "Read GFOC.vi"("error in (no error)"=w8092, "Instrument in"=w8093) -> ("error out"=w8089:errorcluster, "Opt_Continuous.lvclass"=w8091:refnum<class "Opt_Continuous.lvclass">, "Instrument out"=w8087:refnum<class "Instrument.lvclass">)  [unwired: 7 in]
        n3294 = call "Write target.vi"("error in (no error)"=w8089, "target"=w8090, "Optics in"=w8091) -> ("error out"=w8086:errorcluster, "Optics out"=w8088:refnum<class "Opt_Continuous.lvclass">)  [unwired: 7 in]
        n3295 = call "Write GFOC.vi"("error in (no error)"=w8086, "Opt_Continuous.lvclass"=w8088, "Instrument in"=w8087) -> ("error out"=w8083:errorcluster, "Instrument out"=w8085:refnum<class "Instrument.lvclass">)  [unwired: 7 in]
        n3296 = call "Write Instrument.lvclass.vi"("error in (no error)"=w8083, "Instrument.lvclass"=w8085, "S4ACS_GUI in"=w8084) -> ("error out"=w8082:errorcluster, "S4ACS_GUI out"=w8081:refnum<class "S4GUI.lvclass">)  [unwired: 7 in]
      }
      event "GFOC_set": Value Change {
        n3297 = event-data() -> ()  [unwired: 1 in, 4 out]
        n3298 = call "Read Instrument.lvclass.vi"("error in (no error)"=w8114, "S4ACS_GUI in"=w8115) -> ("error out"=w8112:errorcluster, "Instrument.lvclass"=w8113:refnum<class "Instrument.lvclass">, "S4ACS_GUI out"=w8100:refnum<class "S4GUI.lvclass">)  [unwired: 7 in]
        n3299 = call "Read GFOC.vi"("error in (no error)"=w8112, "Instrument in"=w8113) -> ("error out"=w8109:errorcluster, "Opt_Continuous.lvclass"=w8111:refnum<class "Opt_Continuous.lvclass">, "Instrument out"=w8103:refnum<class "Instrument.lvclass">)  [unwired: 7 in]
        n3300 = call-dynamic "Read State Machine.vi"("error in (no error)"=w8109, "Device in"=w8111) -> ("error out"=w8108:errorcluster, "State Machine.lvclass"=w8097:refnum<class "State Machine.lvclass">, "Device out"=w8105:refnum<class "Opt_Continuous.lvclass">)  [unwired: 7 in]
        n3301 = call "Next State.vi"("error in (no error)"=w8108, "New_State"=1, "State Machine in"=w8097) -> ("error out"=w8107:errorcluster, "State Machine out"=w8106:refnum<class "State Machine.lvclass">)  [unwired: 7 in]
        n3302 = call-dynamic "Write State Machine.vi"("error in (no error)"=w8107, "State Machine.lvclass"=w8106, "Device in"=w8105) -> ("error out"=w8102:errorcluster, "Device out"=w8104:refnum<class "Opt_Continuous.lvclass">)  [unwired: 7 in]
        n3303 = call "Write GFOC.vi"("error in (no error)"=w8102, "Opt_Continuous.lvclass"=w8104, "Instrument in"=w8103) -> ("error out"=w8099:errorcluster, "Instrument out"=w8101:refnum<class "Instrument.lvclass">)  [unwired: 7 in]
        n3304 = call "Write Instrument.lvclass.vi"("error in (no error)"=w8099, "Instrument.lvclass"=w8101, "S4ACS_GUI in"=w8100) -> ("error out"=w8098:errorcluster, "S4ACS_GUI out"=w8096:refnum<class "S4GUI.lvclass">)  [unwired: 7 in]
      }
      event "GFOC_stop": Value Change {
        n3305 = event-data() -> ()  [unwired: 1 in, 4 out]
        n3306 = call "Read Instrument.lvclass.vi"("error in (no error)"=w8134, "S4ACS_GUI in"=w8135) -> ("error out"=w8132:errorcluster, "Instrument.lvclass"=w8133:refnum<class "Instrument.lvclass">, "S4ACS_GUI out"=w8119:refnum<class "S4GUI.lvclass">)  [unwired: 7 in]
        n3307 = call "Read GFOC.vi"("error in (no error)"=w8132, "Instrument in"=w8133) -> ("error out"=w8128:errorcluster, "Opt_Continuous.lvclass"=w8131:refnum<class "Opt_Continuous.lvclass">, "Instrument out"=w8122:refnum<class "Instrument.lvclass">)  [unwired: 7 in]
        n3308 = call-dynamic "Read State Machine.vi"("error in (no error)"=w8128, "Device in"=w8131) -> ("error out"=w8127:errorcluster, "State Machine.lvclass"=w8130:refnum<class "State Machine.lvclass">, "Device out"=w8124:refnum<class "Opt_Continuous.lvclass">)  [unwired: 7 in]
        n3309 = call "Next State.vi"("error in (no error)"=w8127, "New_State"=10, "State Machine in"=w8130) -> ("error out"=w8126:errorcluster, "State Machine out"=w8125:refnum<class "State Machine.lvclass">)  [unwired: 7 in]
        n3310 = call-dynamic "Write State Machine.vi"("error in (no error)"=w8126, "State Machine.lvclass"=w8125, "Device in"=w8124) -> ("error out"=w8121:errorcluster, "Device out"=w8123:refnum<class "Opt_Continuous.lvclass">)  [unwired: 7 in]
        n3311 = call "Write GFOC.vi"("error in (no error)"=w8121, "Opt_Continuous.lvclass"=w8123, "Instrument in"=w8122) -> ("error out"=w8118:errorcluster, "Instrument out"=w8120:refnum<class "Instrument.lvclass">)  [unwired: 7 in]
        n3312 = call "Write Instrument.lvclass.vi"("error in (no error)"=w8118, "Instrument.lvclass"=w8120, "S4ACS_GUI in"=w8119) -> ("error out"=w8117:errorcluster, "S4ACS_GUI out"=w8116:refnum<class "S4GUI.lvclass">)  [unwired: 7 in]
      }
      event "GFOC_init": Value Change {
        n3313 = event-data() -> ()  [unwired: 1 in, 4 out]
        n3314 = call "Read Instrument.lvclass.vi"("error in (no error)"=w8154, "S4ACS_GUI in"=w8155) -> ("error out"=w8152:errorcluster, "Instrument.lvclass"=w8153:refnum<class "Instrument.lvclass">, "S4ACS_GUI out"=w8139:refnum<class "S4GUI.lvclass">)  [unwired: 7 in]
        n3315 = call "Read GFOC.vi"("error in (no error)"=w8152, "Instrument in"=w8153) -> ("error out"=w8148:errorcluster, "Opt_Continuous.lvclass"=w8151:refnum<class "Opt_Continuous.lvclass">, "Instrument out"=w8142:refnum<class "Instrument.lvclass">)  [unwired: 7 in]
        n3316 = call-dynamic "Read State Machine.vi"("error in (no error)"=w8148, "Device in"=w8151) -> ("error out"=w8147:errorcluster, "State Machine.lvclass"=w8150:refnum<class "State Machine.lvclass">, "Device out"=w8144:refnum<class "Opt_Continuous.lvclass">)  [unwired: 7 in]
        n3317 = call "Next State.vi"("error in (no error)"=w8147, "New_State"=30, "State Machine in"=w8150) -> ("error out"=w8146:errorcluster, "State Machine out"=w8145:refnum<class "State Machine.lvclass">)  [unwired: 7 in]
        n3318 = call-dynamic "Write State Machine.vi"("error in (no error)"=w8146, "State Machine.lvclass"=w8145, "Device in"=w8144) -> ("error out"=w8141:errorcluster, "Device out"=w8143:refnum<class "Opt_Continuous.lvclass">)  [unwired: 7 in]
        n3319 = call "Write GFOC.vi"("error in (no error)"=w8141, "Opt_Continuous.lvclass"=w8143, "Instrument in"=w8142) -> ("error out"=w8138:errorcluster, "Instrument out"=w8140:refnum<class "Instrument.lvclass">)  [unwired: 7 in]
        n3320 = call "Write Instrument.lvclass.vi"("error in (no error)"=w8138, "Instrument.lvclass"=w8140, "S4ACS_GUI in"=w8139) -> ("error out"=w8137:errorcluster, "S4ACS_GUI out"=w8136:refnum<class "S4GUI.lvclass">)  [unwired: 7 in]
      }
      event "CALW_target": Value Change {
        n3321 = event-data() -> ("NewVal"=w8165:dbl)  [unwired: 1 in, 3 out]
        n3322 = call "Read Instrument.lvclass.vi"("error in (no error)"=w8169, "S4ACS_GUI in"=w8170) -> ("error out"=w8167:errorcluster, "Instrument.lvclass"=w8168:refnum<class "Instrument.lvclass">, "S4ACS_GUI out"=w8159:refnum<class "S4GUI.lvclass">)  [unwired: 7 in]
        n3323 = call "Read CALW.vi"("error in (no error)"=w8167, "Instrument in"=w8168) -> ("error out"=w8164:errorcluster, "Opt_Selector.lvclass"=w8166:refnum<class "Opt_Selector.lvclass">, "Instrument out"=w8162:refnum<class "Instrument.lvclass">)  [unwired: 7 in]
        n3324 = call "Write target.vi"("error in (no error)"=w8164, "target"=w8165, "Optics in"=w8166) -> ("error out"=w8161:errorcluster, "Optics out"=w8163:refnum<class "Opt_Selector.lvclass">)  [unwired: 7 in]
        n3325 = call "Write CALW.vi"("error in (no error)"=w8161, "Opt_Selector.lvclass"=w8163, "Instrument in"=w8162) -> ("error out"=w8158:errorcluster, "Instrument out"=w8160:refnum<class "Instrument.lvclass">)  [unwired: 7 in]
        n3326 = call "Write Instrument.lvclass.vi"("error in (no error)"=w8158, "Instrument.lvclass"=w8160, "S4ACS_GUI in"=w8159) -> ("error out"=w8157:errorcluster, "S4ACS_GUI out"=w8156:refnum<class "S4GUI.lvclass">)  [unwired: 7 in]
      }
      event "CALW_set": Value Change {
        n3327 = event-data() -> ()  [unwired: 1 in, 4 out]
        n3328 = call "Read Instrument.lvclass.vi"("error in (no error)"=w8189, "S4ACS_GUI in"=w8190) -> ("error out"=w8187:errorcluster, "Instrument.lvclass"=w8188:refnum<class "Instrument.lvclass">, "S4ACS_GUI out"=w8175:refnum<class "S4GUI.lvclass">)  [unwired: 7 in]
        n3329 = call "Read CALW.vi"("error in (no error)"=w8187, "Instrument in"=w8188) -> ("error out"=w8184:errorcluster, "Opt_Selector.lvclass"=w8186:refnum<class "Opt_Selector.lvclass">, "Instrument out"=w8178:refnum<class "Instrument.lvclass">)  [unwired: 7 in]
        n3330 = call-dynamic "Read State Machine.vi"("error in (no error)"=w8184, "Device in"=w8186) -> ("error out"=w8183:errorcluster, "State Machine.lvclass"=w8172:refnum<class "State Machine.lvclass">, "Device out"=w8180:refnum<class "Opt_Selector.lvclass">)  [unwired: 7 in]
        n3331 = call "Next State.vi"("error in (no error)"=w8183, "New_State"=1, "State Machine in"=w8172) -> ("error out"=w8182:errorcluster, "State Machine out"=w8181:refnum<class "State Machine.lvclass">)  [unwired: 7 in]
        n3332 = call-dynamic "Write State Machine.vi"("error in (no error)"=w8182, "State Machine.lvclass"=w8181, "Device in"=w8180) -> ("error out"=w8177:errorcluster, "Device out"=w8179:refnum<class "Opt_Selector.lvclass">)  [unwired: 7 in]
        n3333 = call "Write CALW.vi"("error in (no error)"=w8177, "Opt_Selector.lvclass"=w8179, "Instrument in"=w8178) -> ("error out"=w8174:errorcluster, "Instrument out"=w8176:refnum<class "Instrument.lvclass">)  [unwired: 7 in]
        n3334 = call "Write Instrument.lvclass.vi"("error in (no error)"=w8174, "Instrument.lvclass"=w8176, "S4ACS_GUI in"=w8175) -> ("error out"=w8173:errorcluster, "S4ACS_GUI out"=w8171:refnum<class "S4GUI.lvclass">)  [unwired: 7 in]
      }
      event "CALW_stop": Value Change {
        n3335 = event-data() -> ()  [unwired: 1 in, 4 out]
        n3336 = call "Read Instrument.lvclass.vi"("error in (no error)"=w8209, "S4ACS_GUI in"=w8210) -> ("error out"=w8207:errorcluster, "Instrument.lvclass"=w8208:refnum<class "Instrument.lvclass">, "S4ACS_GUI out"=w8194:refnum<class "S4GUI.lvclass">)  [unwired: 7 in]
        n3337 = call "Read CALW.vi"("error in (no error)"=w8207, "Instrument in"=w8208) -> ("error out"=w8203:errorcluster, "Opt_Selector.lvclass"=w8206:refnum<class "Opt_Selector.lvclass">, "Instrument out"=w8197:refnum<class "Instrument.lvclass">)  [unwired: 7 in]
        n3338 = call-dynamic "Read State Machine.vi"("error in (no error)"=w8203, "Device in"=w8206) -> ("error out"=w8202:errorcluster, "State Machine.lvclass"=w8205:refnum<class "State Machine.lvclass">, "Device out"=w8199:refnum<class "Opt_Selector.lvclass">)  [unwired: 7 in]
        n3339 = call "Next State.vi"("error in (no error)"=w8202, "New_State"=10, "State Machine in"=w8205) -> ("error out"=w8201:errorcluster, "State Machine out"=w8200:refnum<class "State Machine.lvclass">)  [unwired: 7 in]
        n3340 = call-dynamic "Write State Machine.vi"("error in (no error)"=w8201, "State Machine.lvclass"=w8200, "Device in"=w8199) -> ("error out"=w8196:errorcluster, "Device out"=w8198:refnum<class "Opt_Selector.lvclass">)  [unwired: 7 in]
        n3341 = call "Write CALW.vi"("error in (no error)"=w8196, "Opt_Selector.lvclass"=w8198, "Instrument in"=w8197) -> ("error out"=w8193:errorcluster, "Instrument out"=w8195:refnum<class "Instrument.lvclass">)  [unwired: 7 in]
        n3342 = call "Write Instrument.lvclass.vi"("error in (no error)"=w8193, "Instrument.lvclass"=w8195, "S4ACS_GUI in"=w8194) -> ("error out"=w8192:errorcluster, "S4ACS_GUI out"=w8191:refnum<class "S4GUI.lvclass">)  [unwired: 7 in]
      }
      event "CALW_init": Value Change {
        n3343 = event-data() -> ()  [unwired: 1 in, 4 out]
        n3344 = call "Read Instrument.lvclass.vi"("error in (no error)"=w8229, "S4ACS_GUI in"=w8230) -> ("error out"=w8227:errorcluster, "Instrument.lvclass"=w8228:refnum<class "Instrument.lvclass">, "S4ACS_GUI out"=w8214:refnum<class "S4GUI.lvclass">)  [unwired: 7 in]
        n3345 = call "Read CALW.vi"("error in (no error)"=w8227, "Instrument in"=w8228) -> ("error out"=w8223:errorcluster, "Opt_Selector.lvclass"=w8226:refnum<class "Opt_Selector.lvclass">, "Instrument out"=w8217:refnum<class "Instrument.lvclass">)  [unwired: 7 in]
        n3346 = call-dynamic "Read State Machine.vi"("error in (no error)"=w8223, "Device in"=w8226) -> ("error out"=w8222:errorcluster, "State Machine.lvclass"=w8225:refnum<class "State Machine.lvclass">, "Device out"=w8219:refnum<class "Opt_Selector.lvclass">)  [unwired: 7 in]
        n3347 = call "Next State.vi"("error in (no error)"=w8222, "New_State"=30, "State Machine in"=w8225) -> ("error out"=w8221:errorcluster, "State Machine out"=w8220:refnum<class "State Machine.lvclass">)  [unwired: 7 in]
        n3348 = call-dynamic "Write State Machine.vi"("error in (no error)"=w8221, "State Machine.lvclass"=w8220, "Device in"=w8219) -> ("error out"=w8216:errorcluster, "Device out"=w8218:refnum<class "Opt_Selector.lvclass">)  [unwired: 7 in]
        n3349 = call "Write CALW.vi"("error in (no error)"=w8216, "Opt_Selector.lvclass"=w8218, "Instrument in"=w8217) -> ("error out"=w8213:errorcluster, "Instrument out"=w8215:refnum<class "Instrument.lvclass">)  [unwired: 7 in]
        n3350 = call "Write Instrument.lvclass.vi"("error in (no error)"=w8213, "Instrument.lvclass"=w8215, "S4ACS_GUI in"=w8214) -> ("error out"=w8212:errorcluster, "S4ACS_GUI out"=w8211:refnum<class "S4GUI.lvclass">)  [unwired: 7 in]
      }
      event "ASEL_target": Value Change {
        n3351 = event-data() -> ("NewVal"=w8240:dbl)  [unwired: 1 in, 3 out]
        n3352 = call "Read Instrument.lvclass.vi"("error in (no error)"=w8244, "S4ACS_GUI in"=w8245) -> ("error out"=w8242:errorcluster, "Instrument.lvclass"=w8243:refnum<class "Instrument.lvclass">, "S4ACS_GUI out"=w8234:refnum<class "S4GUI.lvclass">)  [unwired: 7 in]
        n3353 = call "Read ASEL.vi"("error in (no error)"=w8242, "Instrument in"=w8243) -> ("error out"=w8239:errorcluster, "Opt_Selector.lvclass"=w8241:refnum<class "Opt_Selector.lvclass">, "Instrument out"=w8237:refnum<class "Instrument.lvclass">)  [unwired: 7 in]
        n3354 = call "Write target.vi"("error in (no error)"=w8239, "target"=w8240, "Optics in"=w8241) -> ("error out"=w8236:errorcluster, "Optics out"=w8238:refnum<class "Opt_Selector.lvclass">)  [unwired: 7 in]
        n3355 = call "Write ASEL.vi"("error in (no error)"=w8236, "Opt_Selector.lvclass"=w8238, "Instrument in"=w8237) -> ("error out"=w8233:errorcluster, "Instrument out"=w8235:refnum<class "Instrument.lvclass">)  [unwired: 7 in]
        n3356 = call "Write Instrument.lvclass.vi"("error in (no error)"=w8233, "Instrument.lvclass"=w8235, "S4ACS_GUI in"=w8234) -> ("error out"=w8232:errorcluster, "S4ACS_GUI out"=w8231:refnum<class "S4GUI.lvclass">)  [unwired: 7 in]
      }
      event "ASEL_set": Value Change {
        n3357 = event-data() -> ()  [unwired: 1 in, 4 out]
        n3358 = call "Read Instrument.lvclass.vi"("error in (no error)"=w8264, "S4ACS_GUI in"=w8265) -> ("error out"=w8262:errorcluster, "Instrument.lvclass"=w8263:refnum<class "Instrument.lvclass">, "S4ACS_GUI out"=w8250:refnum<class "S4GUI.lvclass">)  [unwired: 7 in]
        n3359 = call "Read ASEL.vi"("error in (no error)"=w8262, "Instrument in"=w8263) -> ("error out"=w8259:errorcluster, "Opt_Selector.lvclass"=w8261:refnum<class "Opt_Selector.lvclass">, "Instrument out"=w8253:refnum<class "Instrument.lvclass">)  [unwired: 7 in]
        n3360 = call-dynamic "Read State Machine.vi"("error in (no error)"=w8259, "Device in"=w8261) -> ("error out"=w8258:errorcluster, "State Machine.lvclass"=w8247:refnum<class "State Machine.lvclass">, "Device out"=w8255:refnum<class "Opt_Selector.lvclass">)  [unwired: 7 in]
        n3361 = call "Next State.vi"("error in (no error)"=w8258, "New_State"=1, "State Machine in"=w8247) -> ("error out"=w8257:errorcluster, "State Machine out"=w8256:refnum<class "State Machine.lvclass">)  [unwired: 7 in]
        n3362 = call-dynamic "Write State Machine.vi"("error in (no error)"=w8257, "State Machine.lvclass"=w8256, "Device in"=w8255) -> ("error out"=w8252:errorcluster, "Device out"=w8254:refnum<class "Opt_Selector.lvclass">)  [unwired: 7 in]
        n3363 = call "Write ASEL.vi"("error in (no error)"=w8252, "Opt_Selector.lvclass"=w8254, "Instrument in"=w8253) -> ("error out"=w8249:errorcluster, "Instrument out"=w8251:refnum<class "Instrument.lvclass">)  [unwired: 7 in]
        n3364 = call "Write Instrument.lvclass.vi"("error in (no error)"=w8249, "Instrument.lvclass"=w8251, "S4ACS_GUI in"=w8250) -> ("error out"=w8248:errorcluster, "S4ACS_GUI out"=w8246:refnum<class "S4GUI.lvclass">)  [unwired: 7 in]
      }
      event "ASEL_stop": Value Change {
        n3365 = event-data() -> ()  [unwired: 1 in, 4 out]
        n3366 = call "Read Instrument.lvclass.vi"("error in (no error)"=w8284, "S4ACS_GUI in"=w8285) -> ("error out"=w8282:errorcluster, "Instrument.lvclass"=w8283:refnum<class "Instrument.lvclass">, "S4ACS_GUI out"=w8269:refnum<class "S4GUI.lvclass">)  [unwired: 7 in]
        n3367 = call "Read ASEL.vi"("error in (no error)"=w8282, "Instrument in"=w8283) -> ("error out"=w8278:errorcluster, "Opt_Selector.lvclass"=w8281:refnum<class "Opt_Selector.lvclass">, "Instrument out"=w8272:refnum<class "Instrument.lvclass">)  [unwired: 7 in]
        n3368 = call-dynamic "Read State Machine.vi"("error in (no error)"=w8278, "Device in"=w8281) -> ("error out"=w8277:errorcluster, "State Machine.lvclass"=w8280:refnum<class "State Machine.lvclass">, "Device out"=w8274:refnum<class "Opt_Selector.lvclass">)  [unwired: 7 in]
